vi "Wait for state.vi"(8 "error in (no error)":errorcluster, 10 "State":T1=enum."Ready", 11 "FCR Mod ID":i32) -> (0 "error out":errorcluster, 3 "Home?":bool)   [LabVIEW 2020]
uses:
  Newport_FCR100/Libraries/FCR100/Support/Device state -- enum.ctl
  Newport_FCR100/Libraries/FCR100/FCR100.lvlib
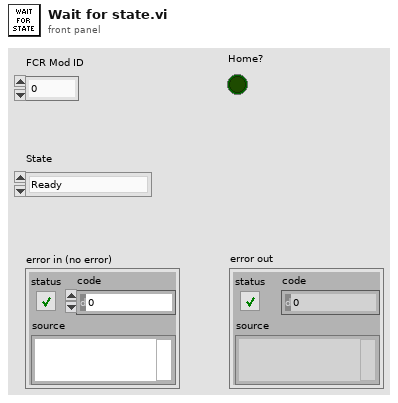
[diagram p1: front panel]
types:
  T1 = typedef "FCR100.lvlib/Device state -- enum.ctl" = enum16{"Not referenced", "Configuration", "Disable", "Ready", "Homing", "Motion"}
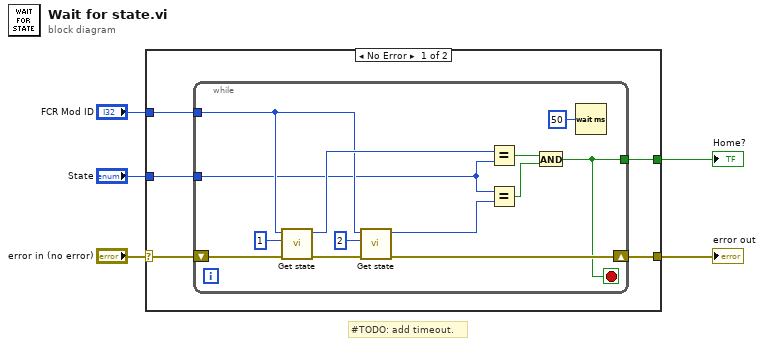
[diagram p0: block diagram]
diagram:
  # "#TODO: add timeout."
  n1 = case shown="No Error" "error in (no error)" {
    selector: "error in (no error)" -> [w9 w24]
    tunnel: "FCR Mod ID" -> [w10 _]
    tunnel: [w8 w24] -> w3
    tunnel: [w7 _] -> w2
    tunnel: "State" -> [w6 _]
    frame No Error {
      n2 = while {
        tunnel: w10 -> [w19]
        tunnel: [w13] -> w7
        shift-right: [w16] -> w8
        shift-left: w9 -> [w17]
        tunnel: w6 -> [w11]
        stop <- w13 stop-if-true
        n3 = call "Get state.vi"("error in"=w17, "Address"=u8 1, "Module ID"=w19) -> ("error out"=w18:errorcluster, "Device state"=w22:T1)  [unwired: 6 in, 1 out]
        n4 = call "Get state.vi"("error in"=w18, "Address"=u8 2, "Module ID"=w19) -> ("error out"=w16:errorcluster, "Device state"=w15:T1)  [unwired: 6 in, 1 out]
        n5 = Equal?(x=w22, y=w11) -> (x = y?=w23:bool)
        n6 = Equal?(x=w11, y=w15) -> (x = y?=w14:bool)
        n7 = And(x=w23, y=w14) -> (x .and. y?=w13:bool)
        n8 = Wait (ms)(milliseconds to wait=u32 50) -> ()  [unwired: 1 out]
      }
    }
    frame Error {
    }
  }
  "error out" <- w3
  "Home?" <- w2
